vi "OccurDetector.vi"(1 "Indice to find":i32, 2 "Reference Matrix":i16[](array[numeric])) -> (0 "Number of occurence":i32)   [LabVIEW 2013]
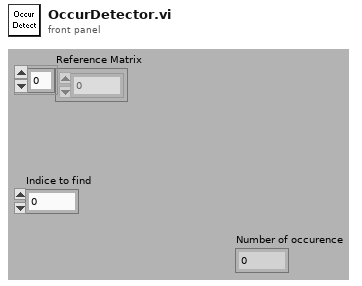
[diagram p1: front panel]
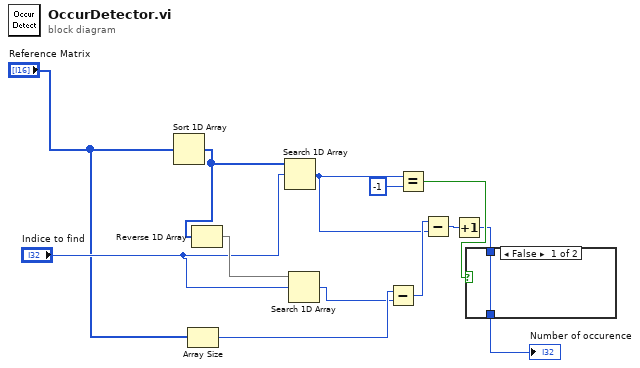
[diagram p0: block diagram]
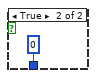
[diagram p2: hidden frame]
diagram:
  n1 = Sort 1D Array(array="Reference Matrix") -> (sorted array=w13:i16[])
  n2 = Array Size(array="Reference Matrix") -> (size(s)=w9:i32)
  n3 = Reverse 1D Array(array=w13) -> (reversed array=w12:i16[])
  n4 = Search 1D Array(1D array=w13, element="Indice to find") -> (index of element=w5:i32)  [unwired: 1 out]
  n5 = Search 1D Array(1D array=w12, element="Indice to find") -> (index of element=w8:i32)  [unwired: 1 out]
  n6 = Subtract(x=w9, y=w8) -> (x-y=w7:i32)
  n7 = Equal?(x=w5, y=-1) -> (x = y?=w3:bool)
  n8 = Subtract(x=w7, y=w5) -> (x-y=w6:i32)
  n9 = Increment(x=w6) -> (x+1=w1:i32)
  n10 = case shown="False" w3 {
    tunnel: [w14 0] -> w2
    tunnel: w1 -> [w14 _]
    frame False {
    }
    frame True {
    }
  }
  "Number of occurence" <- w2
